vi "Read Measurement (Data Rate-Unit Interval).vi"(0 "VISA resource name":refnum<visa-resource-name>, 5 "Channel (1: Channel 1)":i32(ring)=1 items=["Channel 1"=1, "Channel 2"=2, "Channel 3"=3, "Channel 4"=4, "Function 1"=5, "Function 2"=6, "Function 3"=7, "Function 4"=8, "Memory 1"=9, "Memory 2"=10, "Memory 3"=11, "Memory 4"=12], 7 "Measurement (0: Data Rate)":i32(ring) items=["Data Rate", "Unit Interval"], 9 "Maximum Time (10000ms)":u32=10000, 11 "error in (no error)":errorcluster, 12 "Data Rate Type (0: Fully Automatic)":i32(ring) items=["Fully Automatic", "Semi Automatic"], 13 "Data Rate (2.5E9 Hz)":dbl=2500000000.0) -> (4 "VISA resource name out":refnum<visa-resource-name>, 6 "Measurement":dbl, 15 "error out":errorcluster)   [LabVIEW 2012, in "Agilent 8000 Series.lvlib"]
doc: "Initiates, wait for the acquisition to complete and then fetches a Data Rate or Unit Interval measurement."
uses:
  Agilent 8000 Series.lvlib
  Low Level/Fetch Measurement (Data Rate-Unit Interval).vi
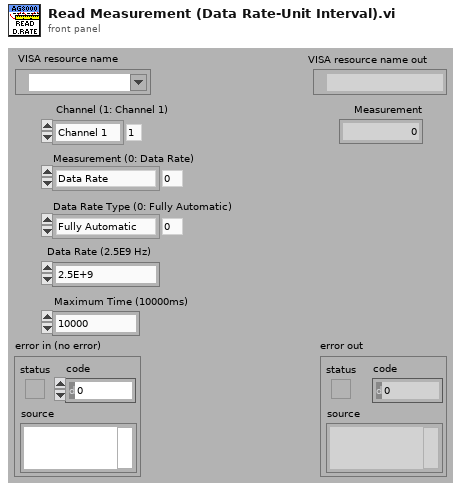
[diagram p1: front panel]
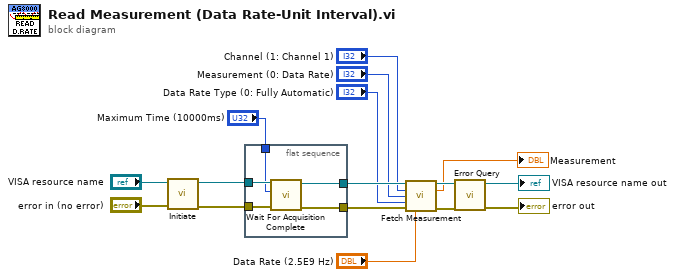
[diagram p0: block diagram]
diagram:
  n1 = call "Initiate.vi"("error in (no error)"="error in (no error)", "VISA resource name"="VISA resource name") -> ("error out"=w13:errorcluster, "VISA resource name out"=w14:refnum<visa-resource-name>)  [unwired: 8 in]
  n2 = flat-sequence {
    tunnel: w14 -> [w21]
    tunnel: w13 -> [w20]
    tunnel: [w19] -> w9
    tunnel: [w18] -> w8
    tunnel: "Maximum Time (10000ms)" -> [w17]
    frame #0 {
      n3 = call "Wait For Acquisition Complete.vi"("error in (no error)"=w20, "Maximum Time (10000ms)"=w17, "VISA resource name"=w21) -> ("error out"=w18:errorcluster, "VISA resource name out"=w19:refnum<visa-resource-name>)  [unwired: 7 in]
    }
  }
  n4 = call-poly "Fetch Measurement.vi"("VISA resource name"=w9, "Channel (1: Channel 1)"="Channel (1: Channel 1)", "Measurement (0: Data Rate)"="Measurement (0: Data Rate)", "Data Rate Type (0: Fully Automatic)"="Data Rate Type (0: Fully Automatic)", "error in (no error)"=w8, "Data Rate (2.5E9 Hz)"="Data Rate (2.5E9 Hz)") -> ("VISA resource name out"=w7:refnum<visa-resource-name>, "Measurement"=→"Measurement":dbl, "error out"=w6:errorcluster)  [unwired: 7 in]
  n5 = call "Error Query.vi"("error in (no error)"=w6, "VISA resource name"=w7) -> ("error out"=→"error out":errorcluster, "VISA resource name out"=→"VISA resource name out":refnum<visa-resource-name>)  [unwired: 6 in, 2 out]
